vi "动子34侧CT内容.vi"() -> (0 "Frist ColData":string, 1 "UpDateData":string[](array[string]), 2 "tablename":string, 3 "UpDateCol":string[](array[string]))   [LabVIEW 2017]
uses:
  Sqlite/CBB/ReadAllData.vi
  Sqlite/SQLite.lvlib
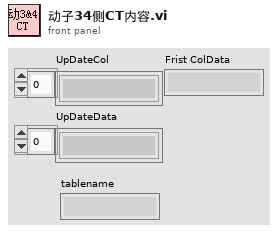
[diagram p1: front panel]
types:
  T1 = typedef "动子3&4CT操作选项.ctl" = enum16{"初始化", "扫码+CheckRoute", "BK拍照", "BT+对位", "RT贴合", "Servo压合", "p400复检", "获取寄存器", "更新等待时间"}
  T2 = typedef "data格式选项.ctl" = enum16{"生成格式", "加载格式"}
  T3 = typedef "缓存操作选项.ctl" = enum16{"初始化", "量测缓存写入", "前侧获取索引", "后侧获取索引", "前侧更新索引", "后侧更新索引", "获取寄存器"}
  T4 = typedef "Data_CT索引操作缓存.ctl" = cluster{"当前data行索引":i32[], "data更新获取索引":T5, "前排提取行号":string, "后排提取行号":string, "当前量测站行号":string, "当前_datetime":string, "量测站操作table缓存":string[], "前排提取_datetime":string, "后排提取_datetime":string}
  T5 = typedef "data更新获取索引.ctl" = cluster{"data更新索引":i32, "前侧获取索引":i32, "后侧获取索引":i32}
  T6 = typedef "表头集合.ctl" = cluster{"product信息":T7, "CT信息":T8, "ER信息":T9, "IOT信息":T10}
  T7 = typedef "product信息.ctl" = cluster{"product表头整合":string[], "量测部分表头":string[], "前侧贴合表头":string[], "后侧贴合表头":string[]}
  T8 = typedef "CT信息.ctl" = cluster{"CT表头整合":string[], "量测CT":string[], "动子1_2CT":string[], "动子3_4CT":string[]}
  T9 = typedef "ER信息.ctl" = cluster{"ER表头整合":string[]}
  T10 = typedef "IOT信息.ctl" = cluster{"IOT表头整合":string[]}
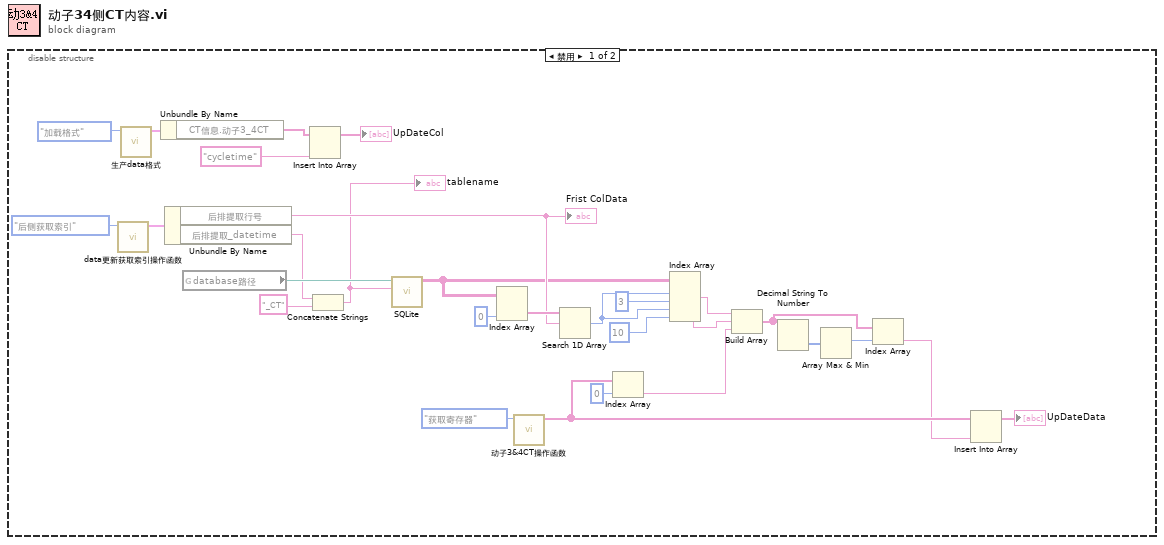
[diagram p0: block diagram]
diagram:
  n1 = disable-structure shown="禁用" {
    frame Disabled {
      n2 = call "data更新获取索引操作函数.vi"("缓存操作选项"=缓存操作选项."后侧获取索引") -> ("Data_CT索引操作缓存"=w28:T4)  [unwired: 9 in, 1 out]
      n3 = call "生产data格式.vi"("data格式选项"=data格式选项."加载格式") -> ("表头格式"=w26:T6)  [unwired: 10 in]
      n4 = Unbundle By Name(w26) -> ("CT信息.动子3_4CT"=w9:string[])
      n5 = Unbundle By Name(w28) -> ("后排提取行号"=w20:string, "后排提取_datetime"=w2:string)
      "Frist ColData" <- w20
      n6 = global read "数据库全局.vi" "database路径"() -> (w24:path)
      n7 = Insert Into Array(array=w9, new element="cycletime") -> (→"UpDateCol":string[])  [unwired: 1 in]
      n8 = Concatenate Strings(w2, "_CT" ("字符串")) -> (w1:string)
      "tablename" <- w1
      n9 = call-poly "SQLite.vi"("Table Name"=w1, "DbPath"=w24) -> ("Results"=w19:string[][])  [unwired: 4 in, 5 out]
      n10 = Index Array(array=w19, index (col)=0 ("禁用的索引 (列)")) -> (element=w21:string[])  [unwired: 1 in]
      n11 = call "动子3&4CT操作函数.vi"("CT操作选项"=动子3&4CT操作选项."获取寄存器") -> ("CT集合"=w6:string[])  [unwired: 8 in, 2 out]
      n12 = Search 1D Array(1D array=w21, element=w20) -> (index of element=w17:i32)  [unwired: 1 in]
      n13 = Index Array(array=w6, index=0 ("索引")) -> (element=w13:string)
      n14 = Index Array(array=w19, index (row) #1=w17, index (col) #1=3 ("禁用的索引 (列)"), index (row) #2=w17, index (col) #2=10 ("禁用的索引 (列)")) -> (element #1=w15:string, element #2=w14:string)
      n15 = Build Array(w15, w14, w13) -> (w11:string[])
      n16 = Decimal String To Number(string=w11) -> (number=w12:i32[])  [unwired: 2 in, 1 out]
      n17 = Array Max & Min(array=w12) -> (max index (indices)=w10:i32)  [unwired: 3 out]
      n18 = Index Array(array=w11, index=w10) -> (element=w5:string)
      n19 = Insert Into Array(array=w6, new element=w5) -> (→"UpDateData":string[])  [unwired: 1 in]
    }
    frame Enabled {
    }
  }
